vi "Tick checker.vi"(3 "Start Sequence":bool, 4 "millisecond timer value":u32) -> (0 "Out":bool, 1 "Sequence time":u32)   [LabVIEW 2018]
uses:
  First Power Up 2018 current/Robot Global Data.vi
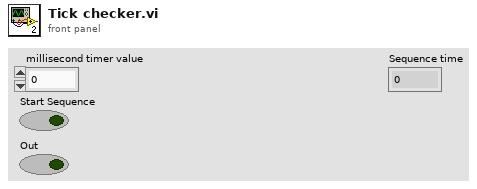
[diagram p1: front panel]
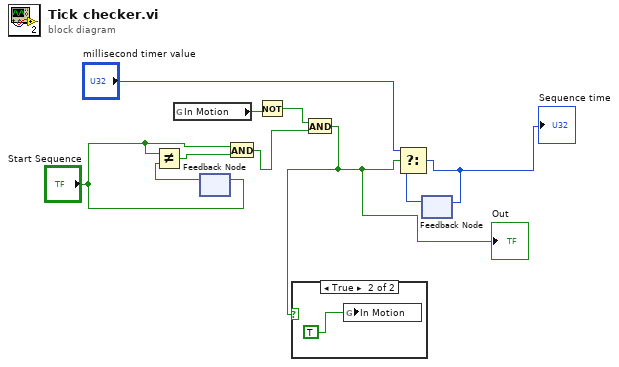
[diagram p0: block diagram]
diagram:
  n1 = global read "Robot Global Data.vi" "In Motion"() -> (w3:bool)
  n2 = feedback #1() -> (w9:bool)  [unwired: 1 in]
  n3 = Not Equal?(x="Start Sequence", y=w9) -> (x != y?=w10:bool)
  n4 = feedback-in #1("Start Sequence") -> ()
  n5 = And(x="Start Sequence", y=w10) -> (x .and. y?=w2:bool)
  n6 = Not(x=w3) -> (.not. x?=w4:bool)
  n7 = And(x=w4, y=w2) -> (x .and. y?=w1:bool)
  "Out" <- w1
  n8 = case shown="True" w1 {
    frame False {
    }
    frame True {
      n9 = global write "Robot Global Data.vi" "In Motion"(TRUE) -> ()
    }
  }
  n10 = feedback #2() -> (w8:u32)  [unwired: 1 in]
  n11 = Select(t="millisecond timer value", s=w1, f=w8) -> (s? t:f=w6:u32)
  "Sequence time" <- w6
  n12 = feedback-in #2(w6) -> ()
